vi "lvBuild.vi"(8 "error in (no error)":errorcluster, 11 "CommandLine":string[](array[string])) -> (0 "error out":errorcluster, 2 "test details":string, 3 "output to action":string)   [LabVIEW 2019]
uses:
  <vilib>/AppBuilder/AB_API_Simple/Build (path).vi
  <vilib>/AppBuilder/AB_API_Simple/NI_App_Builder_API.lvlib
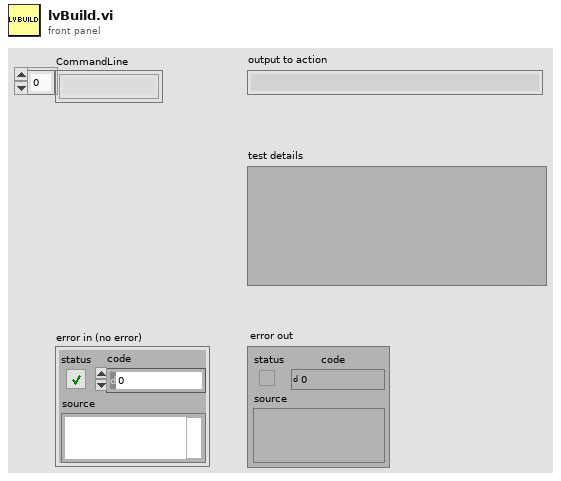
[diagram p1: front panel]
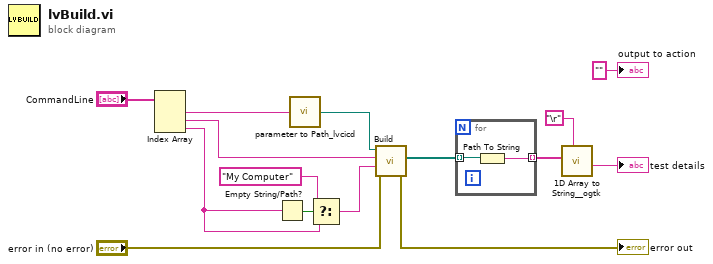
[diagram p0: block diagram]
diagram:
  n1 = Index Array(array="CommandLine") -> (element #1=w6:string, element #2=w12:string, element #3=w3:string)  [unwired: 3 in]
  n2 = Empty String/Path?(string/path=w3) -> (empty?=w5:bool)
  n3 = call "parameter to Path_lvcicd.vi"("String"=w6) -> ("Path"=w7:path)
  n4 = Select(t="My Computer" ("element"), s=w5, f=w3) -> (s? t:f=w2:string)
  n5 = call-poly <vilib>:"Build.vi"("error in (no error)"="error in (no error)", "Name of target (My Computer)"=w2, "Name of build specification (if empty: build all)"=w12, "Path to project"=w7) -> ("error out"=→"error out":errorcluster, "Generated files"=w11:path[])  [unwired: 6 in]
  n6 = for {
    tunnel: w11 -> [w17] mode=indexing
    tunnel: [w16] -> w10 mode=indexing
    n7 = Path To String(path=w17) -> (string=w16:string)
  }
  n8 = call <userlib>:"1D Array to String__ogtk.vi"("delimiter (Tab)"="\r", "Array of Strings"=w10) -> ("delimited string"=→"test details":string)  [unwired: 9 in]
  "output to action" <- "" ("output to action")
